vi "Get All Build Spec Details.vi"(11 "error in (no error)":errorcluster) -> (4 "Build Spec Details":T1[](array[typedef]), 15 "error out":errorcluster)   [LabVIEW 2021, in "Packager Helpers.lvlib"]
uses:
  controls/Build Spec Details.ctl
  <vilib>/AppBuilder/AB_API/common/AB_API Build Object Selector.ctl
  <vilib>/AppBuilder/AB_API/Build/NI_AB_API_Build.lvclass
  Packager Helpers.lvlib
  Dictionary/Dictionary.lvlib
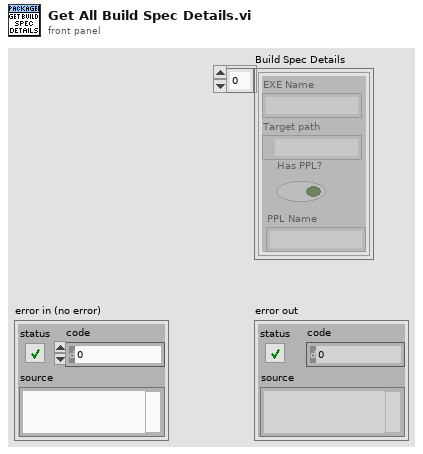
[diagram p1: front panel]
types:
  T1 = typedef "Packager Helpers.lvlib/Build Spec Details.ctl" = cluster{"EXE Name":string, "Target path":path, "Has PPL?":bool, "PPL Name":string}
  T2 = typedef "AB_API Build Object Selector.ctl" = enum16{"Source Distribution", "Deployable Source Distribution", "DLL", "EXE", "Packed Library", "Deployable Packed Library", "RT EXE", ".NET Interop Assembly"}
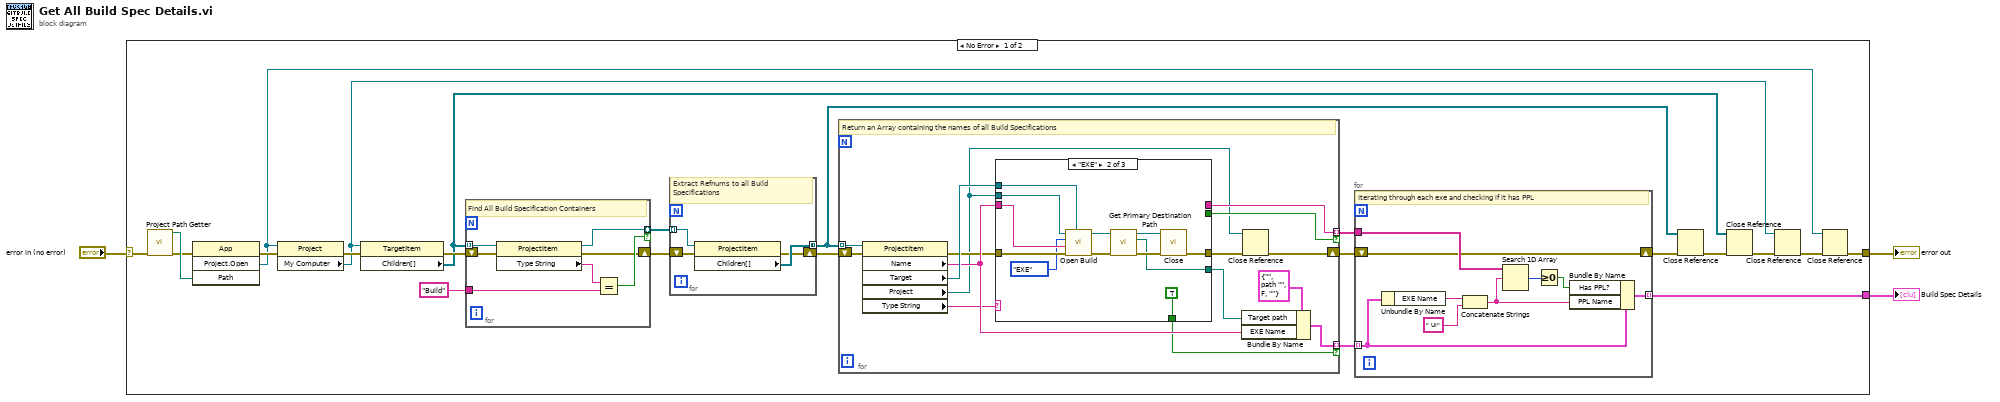
[diagram p0: block diagram]
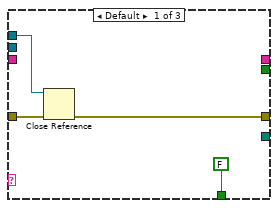
[diagram p2: hidden frame]
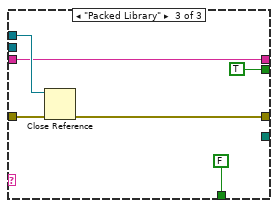
[diagram p3: hidden frame]
diagram:
  n1 = case shown="No Error" "error in (no error)" {
    selector: "error in (no error)" -> [w21 w84]
    tunnel: [w9 w84] -> w3
    tunnel: [w6 _] -> w2
    frame No Error {
      n2 = call "Project Path Getter.vi"("error in (no error)"=w21) -> ("Path"=w22:path, "error out"=w20:errorcluster)  [unwired: 13 in]
      n3 = invoke class="App" method="Project.Open"(error in=w20, "Path"=w22) -> (error out=w19:errorcluster, "Project:Open"=w7:refnum<vi>)  [unwired: 2 in, 2 out]
      n4 = property class="Project"(reference=w7, error in=w19) -> (error out=w18:errorcluster, "My Computer"=w8:refnum<vi>)  [unwired: 1 out]
      n5 = property class="TargetItem"(reference=w8, error in=w18) -> (error out=w17:errorcluster, "Children[]"=w12:refnum<vi>[])  [unwired: 1 out]
      n6 = for {
        tunnel: w12 -> [w74] mode=indexing
        tunnel: [w69] -> w11 mode=indexing if=w73
        shift-right: [w71] -> w26
        shift-left: w17 -> [w72]
        tunnel: "Build" ("y") -> [w68]
        # "Find All Build Specification Containers"
        n7 = property class="ProjectItem"(reference=w74, error in=w72) -> (reference out=w69:refnum<vi>, error out=w71:errorcluster, "Type String"=w70:string)
        n8 = Equal?(x=w70, y=w68) -> (x = y?=w73:bool)
      }
      n9 = for {
        tunnel: w11 -> [w67] mode=indexing
        tunnel: [w66] -> w14 mode=concatenating
        shift-right: [w64] -> w25
        shift-left: w26 -> [w65]
        # "Extract Refnums to all Build Specifications"
        n10 = property class="ProjectItem"(reference=w67, error in=w65) -> (error out=w64:errorcluster, "Children[]"=w66:refnum<vi>[])  [unwired: 1 out]
      }
      n11 = for {
        tunnel: w14 -> [w35] mode=indexing
        shift-right: [w28] -> w24
        shift-left: w25 -> [w39]
        tunnel: [w38] -> w16 mode=indexing if=w34
        tunnel: [w30] -> w4 mode=indexing if=w29
        # "Return an Array containing the names of all Build Specifications"
        n12 = property class="ProjectItem"(reference=w35, error in=w39) -> (error out=w37:errorcluster, "Name"=w40:string, "Target"=w41:refnum<vi>, "Project"=w27:refnum<vi>, "Type String"=w31:string)  [unwired: 1 out]
        n13 = case shown="\"EXE\"" w31 {
          tunnel: [_ w48 _] -> w33
          tunnel: w27 -> [_ w54 _]
          tunnel: w41 -> [w42 w47 w60]
          tunnel: w40 -> [_ w53 w59]
          tunnel: w37 -> [w45 w51 w63]
          tunnel: [w43 w50 w61] -> w36
          tunnel: [FALSE TRUE FALSE] -> w34
          tunnel: [_ _ w59] -> w30
          tunnel: [_ _ TRUE] -> w29
          frame Default {
            n14 = Close Reference(reference=w42, error in (no error)=w45) -> (error out=w43:errorcluster)
          }
          frame "EXE" {
            n15 = call <vilib>:"Open Build.vi"("TargetItem Refnum"=w47, "error in (no error)"=w51, "Build specification name"=w53, "Build object selector"=AB_API_Build_Object_Selector."EXE", "Project Refnum"=w54) -> ("error out"=w52:errorcluster, "NI_AB_API_Build out"=w55:refnum<class "NI_AB_API_Build.lvclass">)  [unwired: 5 in]
            n16 = call-dynamic "Get Primary Destination Path.vi"("error in (no error)"=w52, "NI_AB_API_Build in"=w55) -> ("error out"=w57:errorcluster, "Primary destination path"=w48:path, "NI_AB_API_Build out"=w56:refnum<class "NI_AB_API_Build.lvclass">)  [unwired: 7 in]
            n17 = call-dynamic "Close.vi"("error in (no error)"=w57, "NI_AB_API_Build in"=w56) -> ("error out"=w50:errorcluster)  [unwired: 9 in]
          }
          frame "Packed Library" {
            n18 = Close Reference(reference=w60, error in (no error)=w63) -> (error out=w61:errorcluster)
          }
        }
        n19 = Bundle By Name(cluster=T1 {"EXE Name"="", "Target path"=path "", "Has PPL?"=FALSE, "PPL Name"=""}, "Target path"=w33, "EXE Name"=w40) -> (w38:T1)
        n20 = Close Reference(reference=w27, error in (no error)=w36) -> (error out=w28:errorcluster)
      }
      n21 = for {
        tunnel: w4 -> [w82]
        shift-right: [w76] -> w23
        shift-left: w24 -> [w76]
        tunnel: w16 -> [w79] mode=indexing
        tunnel: [w75] -> w6 mode=indexing
        # "Iterating through each exe and checking if it has PPL"
        n22 = Unbundle By Name(w79) -> ("EXE Name"=w83:string)
        n23 = Concatenate Strings(w83, " UI" ("string")) -> (w77:string)
        n24 = Search 1D Array(1D array=w82, element=w77) -> (index of element=w81:i32)  [unwired: 1 in]
        n25 = Greater Or Equal To 0?(x=w81) -> (x >= 0?=w80:bool)
        n26 = Bundle By Name(cluster=w79, "Has PPL?"=w80, "PPL Name"=w77) -> (w75:T1)
      }
      n27 = Close Reference(reference=w14, error in (no error)=w23) -> (error out=w15:errorcluster)
      n28 = Close Reference(reference=w12, error in (no error)=w15) -> (error out=w13:errorcluster)
      n29 = Close Reference(reference=w8, error in (no error)=w13) -> (error out=w10:errorcluster)
      n30 = Close Reference(reference=w7, error in (no error)=w10) -> (error out=w9:errorcluster)
    }
    frame Error {
    }
  }
  "error out" <- w3
  "Build Spec Details" <- w2
